vi "RP calculate subset.vi"(5 "Samples per trigger increment":i32=2, 6 "Round off":i32=4096 format="0x%x (%d)", 7 "RAM size":i32=268435456 format="0x%x (%d)", 8 "Trigger start position":i32, 9 "Pre-trigger samples":i32=100000 format="0x%x (%d)", 10 "Bytes per sample":i32, 11 "Post-trigger samples":i32 format="0x%x (%d)") -> (0 "Merged subsets":u64[](array[numeric]) format="0x%x (%d)", 1 "record length":i32 format="0x%x (%d)", 2 "pre-trigger trim":i32, 3 "Subsets":i32[][](array[numeric]) format="0x%x (%d)")   [LabVIEW 2024]
uses:
  Mode.ctl
panel:
  out "post-trigger trim":i32
  out "subset end":i32 format="0x%x (%d)"
  out "subset start":i32 format="0x%x (%d)"
  in  "Mode":T1=enum."Digitizer"
  # "ends"
  # "starts"
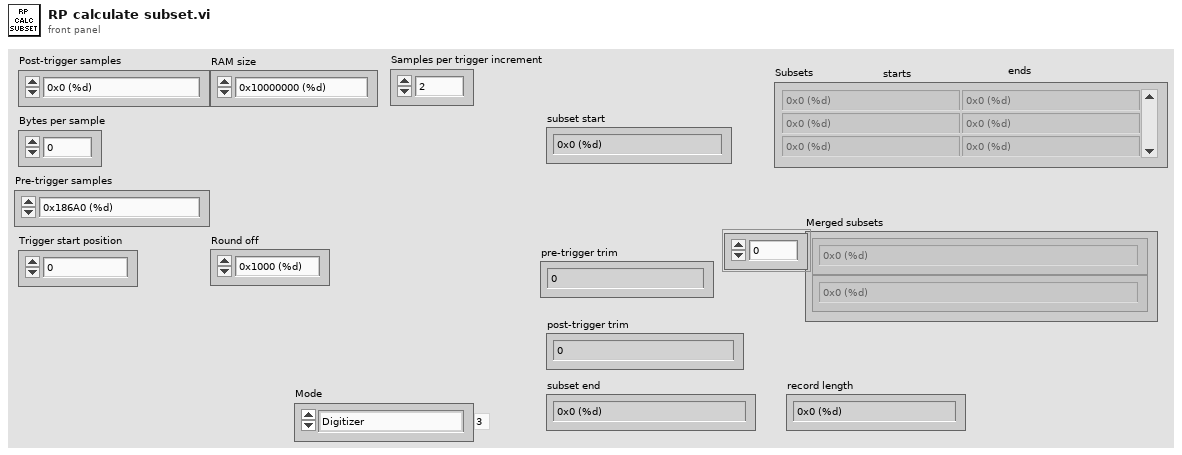
[diagram p1: front panel]
types:
  T1 = typedef "Mode.ctl" = enum16{"Filter", "Lockin test", "Snapshot test", "Digitizer", "Current-Voltage"}
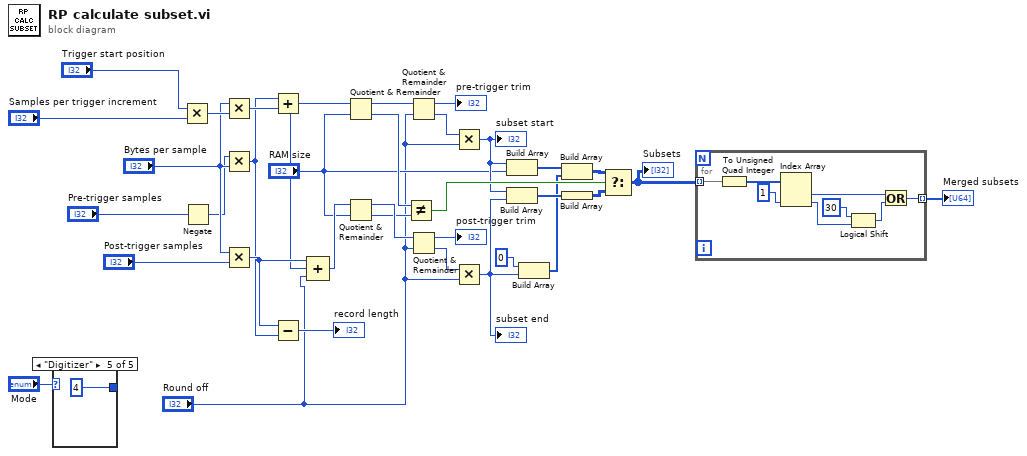
[diagram p0: block diagram]
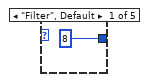
[diagram p2: hidden frame]
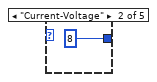
[diagram p3: hidden frame]
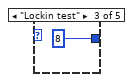
[diagram p4: hidden frame]
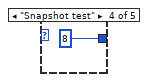
[diagram p5: hidden frame]
diagram:
  n1 = case shown="\"Digitizer\"" "Mode" {
    tunnel: [8 8 8 8 4] -> _
    frame "Filter", Default {
    }
    frame "Current-Voltage" {
    }
    frame "Lockin test" {
    }
    frame "Snapshot test" {
    }
    frame "Digitizer" {
    }
  }
  n2 = Multiply(x="Trigger start position", y="Samples per trigger increment") -> (x*y=w6:i32)
  n3 = Negate(x="Pre-trigger samples") -> (-x=w2:i32)
  n4 = Multiply(x="Bytes per sample", y=w6) -> (x*y=w11:i32)
  n5 = Multiply(x=w2, y="Bytes per sample") -> (x*y=w10:i32)
  n6 = Multiply(x="Bytes per sample", y="Post-trigger samples") -> (x*y=w12:i32)
  n7 = Add(x=w10, y=w11) -> (x+y=w31:i32)
  n8 = Subtract(x=w12, y=w10) -> (x-y=→"record length":i32)
  n9 = Compound Arithmetic op=ADD(w12, w11, "Round off") -> (w33:i32)
  n10 = Quotient & Remainder(x=w31, y="RAM size") -> (x-y*floor(x/y)=w30:i32, floor(x/y)=w25:i32)
  n11 = Quotient & Remainder(x=w33, y="RAM size") -> (x-y*floor(x/y)=w32:i32, floor(x/y)=w24:i32)
  n12 = Not Equal?(x=w25, y=w24) -> (x != y?=w22:bool)
  n13 = Quotient & Remainder(x=w30, y="Round off") -> (x-y*floor(x/y)=→"pre-trigger trim":i32, floor(x/y)=w29:i32)
  n14 = Quotient & Remainder(x=w32, y="Round off") -> (x-y*floor(x/y)=→"post-trigger trim":i32, floor(x/y)=w28:i32)
  n15 = Multiply(x=w29, y="Round off") -> (x*y=w20:i32)
  "subset start" <- w20
  n16 = Multiply(x=w28, y="Round off") -> (x*y=w18:i32)
  "subset end" <- w18
  n17 = Build Array(w20, "RAM size") -> (w16:i32[])
  n18 = Build Array(w20, w18) -> (w23:i32[])
  n19 = Build Array(0 ("element"), w18) -> (w15:i32[])
  n20 = Build Array(w16, w15) -> (w14:i32[][])
  n21 = Build Array(w23) -> (w21:i32[][])
  n22 = Select(t=w14, s=w22, f=w21) -> (s? t:f=w8:i32[][])
  "Subsets" <- w8
  n23 = for {
    tunnel: w8 -> [w48] mode=indexing
    tunnel: [w41] -> w7 mode=indexing
    n24 = To Unsigned Quad Integer(1:w48) -> (0:w47:u64[])
    n25 = Index Array(array=w47, index #2=1 ("index")) -> (element #1=w43:u64, element #2=w45:u64)  [unwired: 1 in]
    n26 = Logical Shift(y=i16 30, x=w45) -> (x << y=w42:u64)
    n27 = Or(x=w43, y=w42) -> (x .or. y?=w41:u64)
  }
  "Merged subsets" <- w7
